vi "RemoteDCPowerSession_CallCloseMeasurementLinkSessionWithCloseBehavior_RemoteSessionClosed.vi"(8 "error in (no error)":errorcluster) -> (0 "error out":errorcluster, 2 "result":string, 3 "pass":bool)   [LabVIEW 2020, in "MeasurementServerTests.lvlib"]
uses:
  MeasurementServerTests.lvlib
  Runtime/MeasurementLink niDCPower/Instrument/Instrument.lvclass
  Runtime/MeasurementLink Instrument/IInstrument/Close Session Behavior.ctl
  Runtime/MeasurementLink Instrument/IInstrument/IInstrument.lvclass
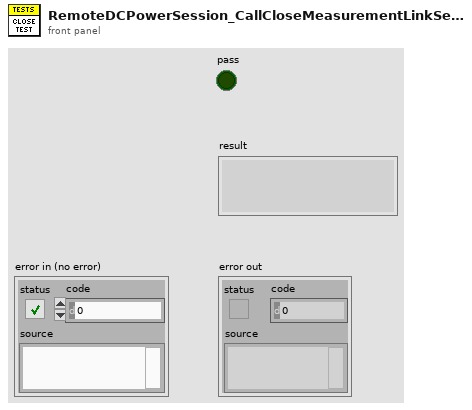
[diagram p1: front panel]
types:
  T1 = typedef "MeasurementLink Instrument.lvlib/IInstrument.lvclass/Close Session Behavior.ctl" = enum16{"Close Session", "Detach Session"}
  T2 = typedef "MeasurementLink Instrument.lvlib/IInstrument.lvclass/Remote Connection Options.ctl" = cluster{"session name":string, "address":string, "port":u32}
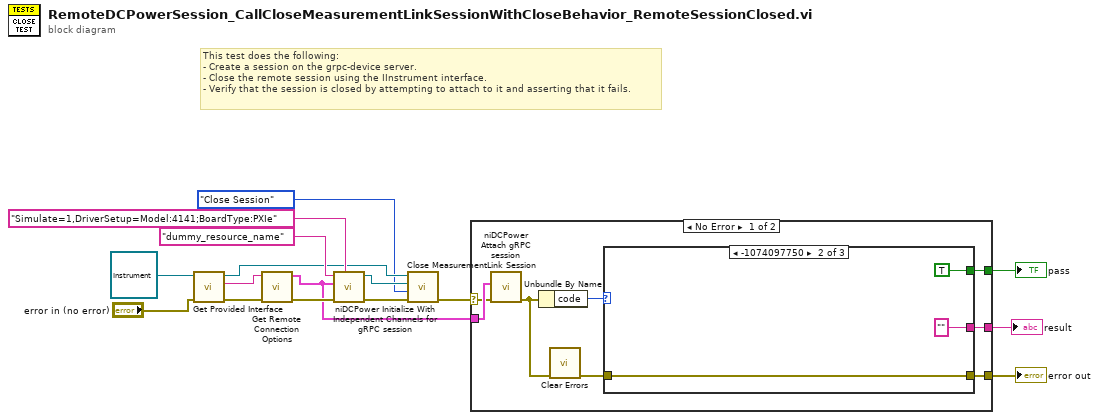
[diagram p0: block diagram]
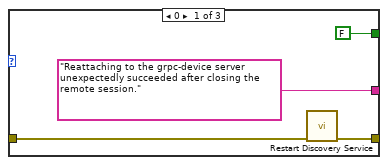
[diagram p2: hidden frame]
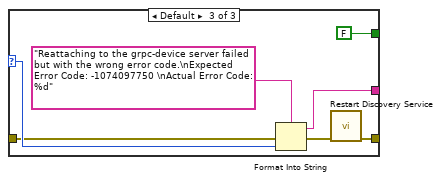
[diagram p3: hidden frame]
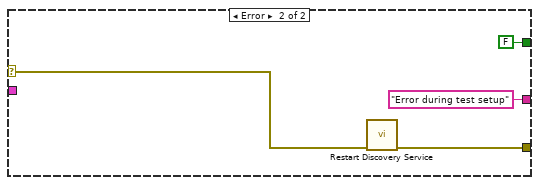
[diagram p4: hidden frame]
diagram:
  # "This test does the following:\n- Create a session on the grpc-device server.\n- Close the remote session using the IInstrument interface.\n- Verify that the session is closed by attempting to attach to it and asserting that it fails."
  n1 = call-dynamic "Get Provided Interface.vi"("error in (no error)"="error in (no error)", "instrument in"=refnum<class "Instrument.lvclass"> refnum ("MeasurementLink niDCPower.lvlib:Instrument.lvclass")) -> ("error out"=w13:errorcluster, "provided interface"=w12:string, "instrument out"=w9:refnum<class "Instrument.lvclass">)  [unwired: 7 in]
  n2 = call "Get Remote Connection Options.vi"("error in (no error)"=w13, "provided interface"=w12) -> ("error out"=w15:errorcluster, "remote connection options"=w6:T2)  [unwired: 8 in]
  n3 = call <instrlib>:"niDCPower Initialize With Independent Channels for gRPC session.vi"("option string"="Simulate=1,DriverSetup=Model:4141;BoardType:PXIe", "error in (no error)"=w15, "gRPC options"=w6, "resource name"="dummy_resource_name") -> ("error out"=w10:errorcluster, "instrument handle out"=w8:refnum<k15>)  [unwired: 6 in]
  n4 = call-dynamic "Close MeasurementLink Session.vi"("error in (no error)"=w10, "close session behavior"=Close_Session_Behavior."Close Session", "session in"=w8, "instrument in"=w9) -> ("error out"=w4:errorcluster)  [unwired: 7 in]
  n5 = case shown="No Error" w4 {
    selector: w4 -> [w23 w40]
    tunnel: w6 -> [w24 _]
    tunnel: [w18 w39] -> w3
    tunnel: [w22 FALSE] -> w2
    tunnel: [w17 "Error during test setup" ("f")] -> w1
    frame No Error {
      n6 = call <instrlib>:"niDCPower Attach gRPC session.vi"("error in (no error)"=w23, "gRPC options"=w24) -> ("error out"=w20:errorcluster)  [unwired: 8 in, 1 out]
      n7 = Unbundle By Name(w20) -> ("code"=w21:i32)
      n8 = call <vilib>:"Clear Errors.vi"("error in (no error)"=w20) -> ("error out"=w19:errorcluster)  [unwired: 5 in, 1 out]
      n9 = case shown="-1074097750" w21 {
        selector: w21 -> [_ _ w37]
        tunnel: ["Reattaching to the grpc-device server unexpectedly succeeded after closing the remote session." ("f") "" ("f") w36] -> w17
        tunnel: [FALSE TRUE FALSE] -> w22
        tunnel: w19 -> [w26 w29 w34]
        tunnel: [w25 w29 w32] -> w18
        frame 0 {
          n10 = call "Restart Discovery Service.vi"("error in"=w26) -> ("error out"=w25:errorcluster)  [unwired: 10 in]
        }
        frame -1074097750 {
        }
        frame Default {
          n11 = Format Into String(format string="Reattaching to the grpc-device server failed but with the wrong error code.\nExpected Error Code: -1074097750 \nActual Error Code: %d" ("f"), error in=w34, w37) -> (resulting string=w36:string, error out=w33:errorcluster)  [unwired: 1 in]
          n12 = call "Restart Discovery Service.vi"("error in"=w33) -> ("error out"=w32:errorcluster)  [unwired: 10 in]
        }
      }
    }
    frame Error {
      n13 = call "Restart Discovery Service.vi"("error in"=w40) -> ("error out"=w39:errorcluster)  [unwired: 10 in]
    }
  }
  "error out" <- w3
  "pass" <- w2
  "result" <- w1
